vi "Array Generation.vi"   [LabVIEW 2020, in "Tests.lvlib"]
uses:
  Tests.lvlib
  aaaa630d-7f0e-475b-802a-d37130267d70.vi
  5ca72616-822f-4046-9a80-c5ab2972504e.vi
  4853ee72-4ff1-4d6a-b14f-368f37e279dd.vi
  e07fba94-1f70-4b86-84c6-d3476923f867.vi
  4e081e4f-5d74-4334-bd3a-36c1155a11f6.vi
  51eb5084-1d0a-43bd-aa82-86afa92a1daa.vi
  2885857f-a0cf-4198-a612-bb3ca9208936.vi
  bb39d310-558e-451e-8b95-db3bf09071d7.vi
  <vilib>/dlg_ctls.llb/Space Constant.vi
  aaaa630d-7f0e-475b-802a-d37130267d70.vi/b24c019a-0099-4d06-9010-75d0c3ff117b.vi
  5ca72616-822f-4046-9a80-c5ab2972504e.vi/b24c019a-0099-4d06-9010-75d0c3ff117b.vi
  4853ee72-4ff1-4d6a-b14f-368f37e279dd.vi/b24c019a-0099-4d06-9010-75d0c3ff117b.vi
  e07fba94-1f70-4b86-84c6-d3476923f867.vi/b24c019a-0099-4d06-9010-75d0c3ff117b.vi
  4e081e4f-5d74-4334-bd3a-36c1155a11f6.vi/48c7ac7e-bb0d-49e2-af2c-796dbdcbcaf5.vi
  51eb5084-1d0a-43bd-aa82-86afa92a1daa.vi/48c7ac7e-bb0d-49e2-af2c-796dbdcbcaf5.vi
  2885857f-a0cf-4198-a612-bb3ca9208936.vi/48c7ac7e-bb0d-49e2-af2c-796dbdcbcaf5.vi
  bb39d310-558e-451e-8b95-db3bf09071d7.vi/48c7ac7e-bb0d-49e2-af2c-796dbdcbcaf5.vi
  <vilib>/addons/_JKI Toolkits/Caraya/classes/Assert/Assert Equal Value_Variant.vi
  <vilib>/addons/_JKI Toolkits/Caraya/classes/Assert/Assert.lvclass
  <vilib>/addons/_JKI Toolkits/Caraya/classes/Test/Test.lvclass
types:
  T1 = cluster{"Expression":string, "Array":dbl[], "Array":dbl[]}
  T2 = cluster{"Expression":string, "Array":dbl[], "Array":dbl[]}[]
  T3 = cluster{"Expression":string, "Array":i32[], "Array":i32[]}
  T4 = cluster{"Expression":string, "Array":i32[], "Array":i32[]}[]
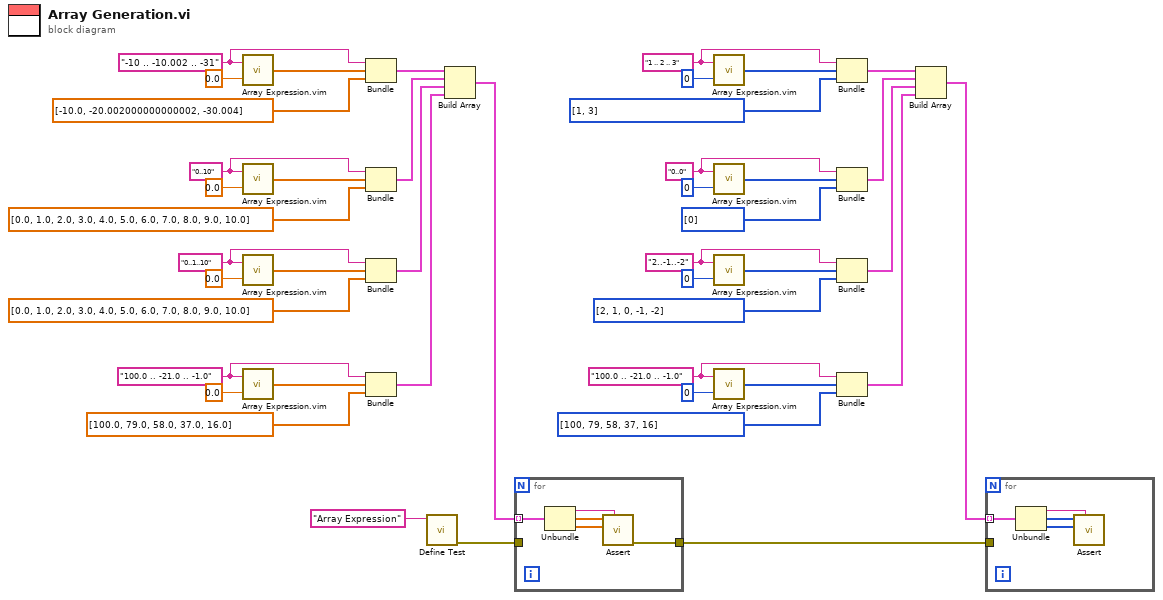
[diagram p0: block diagram]
diagram:
  w1 = "100.0 .. -21.0 .. -1.0" ("Expression")
  w2 = "2..-1..-2" ("Expression")
  w3 = "0..0" ("Expression")
  w4 = "1 .. 2 .. 3" ("Expression")
  w27 = "100.0 .. -21.0 .. -1.0" ("Expression")
  w29 = "0..1..10" ("Expression")
  w30 = "0..10" ("Expression")
  w38 = "-10 .. -10.002 .. -31" ("Expression")
  n1 = call "Array Expression.vim"("Type"=0.0, "Expression"=w38) -> ("Array"=w42:dbl[])
  n2 = call "Array Expression.vim"("Type"=0.0, "Expression"=w30) -> ("Array"=w36:dbl[])
  n3 = call "Array Expression.vim"("Type"=0.0, "Expression"=w29) -> ("Array"=w32:dbl[])
  n4 = call "Array Expression.vim"("Type"=0.0, "Expression"=w27) -> ("Array"=w25:dbl[])
  n5 = Bundle("Expression"=w38, "Array"=w42, "Array"=dbl[] [-10.0, -20.002000000000002, -30.004]) -> (w40:T1)  [unwired: 1 in]
  n6 = Bundle("Expression"=w30, "Array"=w36, "Array"=dbl[] [0.0, 1.0, 2.0, 3.0, 4.0, 5.0, 6.0, 7.0, 8.0, 9.0, 10.0]) -> (w34:T1)  [unwired: 1 in]
  n7 = Bundle("Expression"=w29, "Array"=w32, "Array"=dbl[] [0.0, 1.0, 2.0, 3.0, 4.0, 5.0, 6.0, 7.0, 8.0, 9.0, 10.0]) -> (w28:T1)  [unwired: 1 in]
  n8 = Bundle("Expression"=w27, "Array"=w25, "Array"=dbl[] [100.0, 79.0, 58.0, 37.0, 16.0]) -> (w23:T1)  [unwired: 1 in]
  n9 = call <vilib>:"Define Test.vi"("Label (VI Title)"="Array Expression") -> ("error out"=w43:errorcluster)  [unwired: 10 in]
  n10 = Build Array(w40, w34, w28, w23) -> (w39:T2)
  n11 = for {
    tunnel: w39 -> [w50] mode=indexing
    tunnel: w43 -> [_]
    tunnel: [w46] -> w5
    n12 = Unbundle(w50) -> ("Expression"=w47:string, "Array"=w49:dbl[], "Array"=w48:dbl[])
    n13 = call-poly <vilib>:"Assert.vi"("Label"=w47, "Y"=w48, "X"=w49) -> ("error out"=w46:errorcluster)  [unwired: 8 in]
  }
  n14 = call "Array Expression.vim"("Type"=0, "Expression"=w4) -> ("Array"=w7:i32[])
  n15 = call "Array Expression.vim"("Type"=0, "Expression"=w3) -> ("Array"=w12:i32[])
  n16 = call "Array Expression.vim"("Type"=0, "Expression"=w2) -> ("Array"=w16:i32[])
  n17 = call "Array Expression.vim"("Type"=0, "Expression"=w1) -> ("Array"=w20:i32[])
  n18 = Bundle("Expression"=w4, "Array"=w7, "Array"=i32[] [1, 3]) -> (w9:T3)  [unwired: 1 in]
  n19 = Bundle("Expression"=w3, "Array"=w12, "Array"=i32[] [0]) -> (w14:T3)  [unwired: 1 in]
  n20 = Bundle("Expression"=w2, "Array"=w16, "Array"=i32[] [2, 1, 0, -1, -2]) -> (w18:T3)  [unwired: 1 in]
  n21 = Bundle("Expression"=w1, "Array"=w20, "Array"=i32[] [100, 79, 58, 37, 16]) -> (w22:T3)  [unwired: 1 in]
  n22 = Build Array(w9, w14, w18, w22) -> (w10:T4)
  n23 = for {
    tunnel: w10 -> [w54] mode=indexing
    tunnel: w5 -> [_]
    n24 = Unbundle(w54) -> ("Expression"=w51:string, "Array"=w53:i32[], "Array"=w52:i32[])
    n25 = call-poly <vilib>:"Assert.vi"("Label"=w51, "Y"=w52, "X"=w53) -> ()  [unwired: 8 in, 1 out]
  }
